vi "FTW-Logger-NewLog.vi"(0 "FTW Logger Connector":refnum<class "FTW-Logger.lvclass">, 11 "error in":errorcluster) -> (4 "FTW Logger Connector out":refnum<class "FTW-Logger.lvclass">, 6 "New Log File":path, 15 "error out":errorcluster)   [LabVIEW 2015, in "FTW-Logger.lvclass"]
doc: "This method queues an event to be logged by the Logger associated with the LoggerID."
uses:
  FTW-Logger.lvclass
  Connector/FTW-ActorConnector.lvclass
panel:
  # "Inputs"
  # "Outputs"
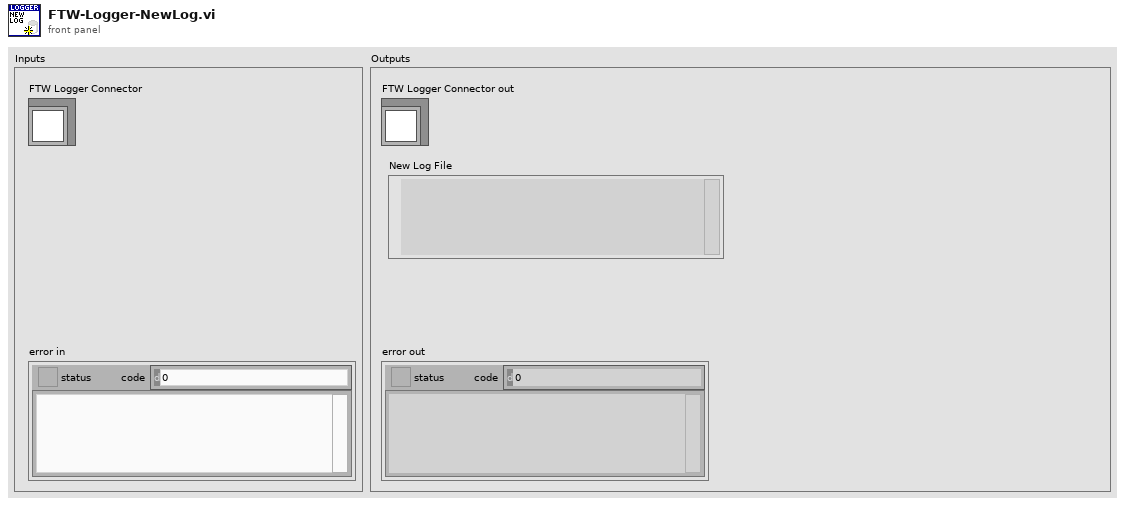
[diagram p1: front panel]
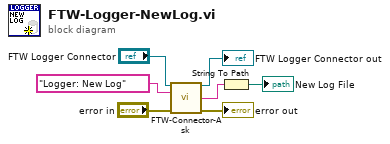
[diagram p0: block diagram]
diagram:
  n1 = call "FTW-Connector-Ask.vi"("FTW Actor Connector"="FTW Logger Connector", "Request Header"="Logger: New Log", "error in"="error in") -> ("FTW Actor Connector out"=→"FTW Logger Connector out":refnum<class "FTW-Logger.lvclass">, "Response Body"=w2:string, "error out"=→"error out":errorcluster)  [unwired: 7 in, 3 out]
  n2 = String To Path(string=w2) -> (path=→"New Log File":path)
